vi "Find API Tester Path.vi"(8 "error in":errorcluster, 11 "DQMH Library Ref":refnum<vi>) -> (0 "error out":errorcluster, 3 "API Tester Path":path)   [LabVIEW 2019, in "Panther Dashboard.lvlib"]
uses:
  Panther Dashboard.lvlib
  <vilib>/Utility/error.llb/Error Cluster From Error Code.vi
  <vilib>/ErrorRing/Error Ring.xnode
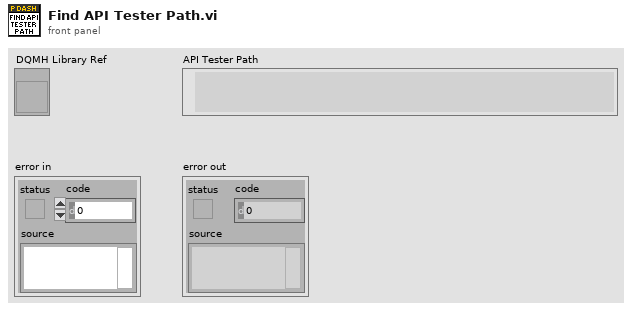
[diagram p1: front panel]
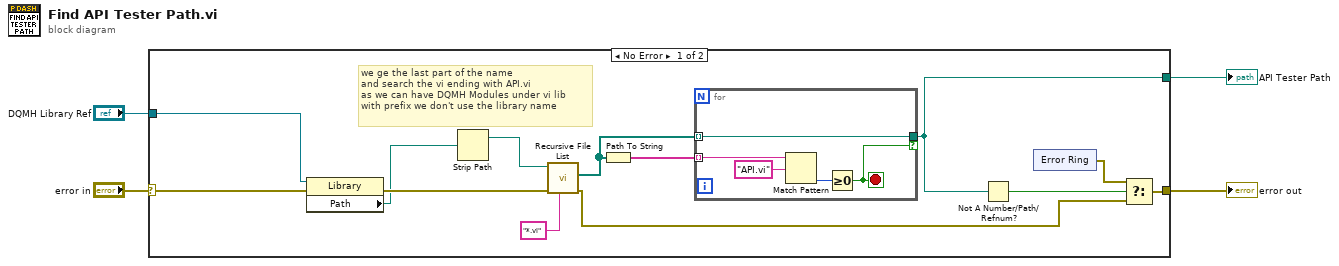
[diagram p0: block diagram]
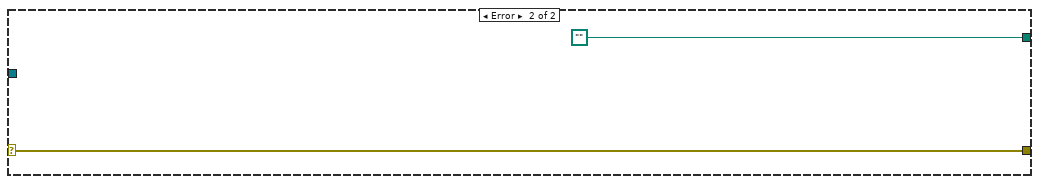
[diagram p2: hidden frame]
diagram:
  n1 = case shown="No Error" "error in" {
    selector: "error in" -> [w13 w29]
    tunnel: [w7 path ""] -> w2
    tunnel: [w15 w29] -> w3
    tunnel: "DQMH Library Ref" -> [w8 _]
    frame No Error {
      # "we ge the last part of the name\nand search the vi ending with API.vi\nas we can have DQMH Modules under vi lib\nwith prefix we don't use the library name"
      n2 = property class="Library"(reference=w8, error in=w13) -> (error out=w14:errorcluster, "Path"=w9:path)  [unwired: 1 out]
      n3 = Strip Path(path=w9) -> (stripped path=w10:path)  [unwired: 1 out]
      n4 = call <vilib>:"Recursive File List.vi"("pattern"="*.vi", "error in (no error)"=w14, "Folder Path"=w10) -> ("error out"=w16:errorcluster, "All Files in Dir"=w11:path[])  [unwired: 4 in, 3 out]
      n5 = Path To String(path=w11) -> (string=w5:string[])
      n6 = for {
        tunnel: w5 -> [w25] mode=indexing
        tunnel: w11 -> [w27] mode=indexing
        tunnel: [w27] -> w7 if=w23
        stop <- w23 stop-if-true
        n7 = Match Pattern(string=w25, regular expression="API.vi") -> (offset past match=w24:i32)  [unwired: 1 in, 3 out]
        n8 = Greater Or Equal To 0?(x=w24) -> (x >= 0?=w23:bool)
      }
      n9 = Not A Number/Path/Refnum?(number/path/refnum=w7) -> (NaN/Path/Refnum?=w6:bool)
      n10 = xnode "Error Ring"() -> ("error out"=w17:errorcluster)
      n11 = Select(t=w17, s=w6, f=w16) -> (s? t:f=w15:errorcluster)
    }
    frame Error {
    }
  }
  "API Tester Path" <- w2
  "error out" <- w3
